vi "Read.vi"(7 "nonEmpty":refnum<k4>, 8 "element in":T3, 10 "parms in":T2={"subchannel"=0, "size (0)"=0, "abort (F)"=FALSE, "timeout"=-1, "ack id (0)"=0, "last elt? (F)"=FALSE, "valid? (T)"=FALSE, "GUID"=""}, 11 "MessengerMCPU in":refnum<class "MessengerMCPU.lvclass">) -> (0 "element out":T3, 1 "wait":bool, 2 "parms out":T1, 3 "MessengerMCPU out":refnum<class "MessengerMCPU.lvclass">)   [LabVIEW 2019, in "MessengerM.lvlib" / "MessengerMCPU.lvclass"]
uses:
  MessengerMCPU.lvclass
  ParmsOut.ctl
  MessengerM.lvlib
  SubChannelCPU/SubChannelCPU.lvclass
  Element.ctl
  ParmsIn.ctl
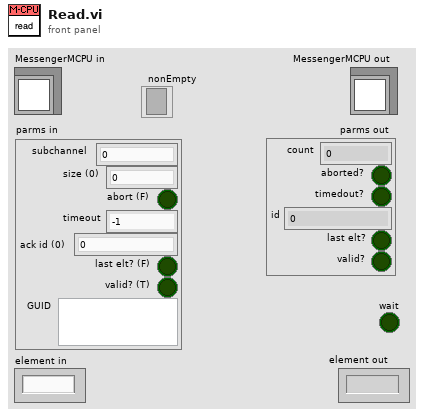
[diagram p1: front panel]
types:
  T1 = typedef "MessengerM.lvlib/ParmsOut.ctl" = cluster{"count":i32, "aborted?":bool, "timedout?":bool, "id":u32, "last elt?":bool, "valid?":bool}
  T2 = typedef "MessengerM.lvlib/ParmsIn.ctl" = cluster{"subchannel":i32, "size (0)":i32, "abort (F)":bool, "timeout":i32, "ack id (0)":u32, "last elt? (F)":bool, "valid? (T)":bool, "GUID":string}
  T3 = typedef "MessengerM.lvlib/Element.ctl" = string
  T4 = cluster{"GUID":string, "sub":refnum<class "SubChannelCPU.lvclass">}[]
  T5 = cluster{"GUID":string, "sub":refnum<class "SubChannelCPU.lvclass">}
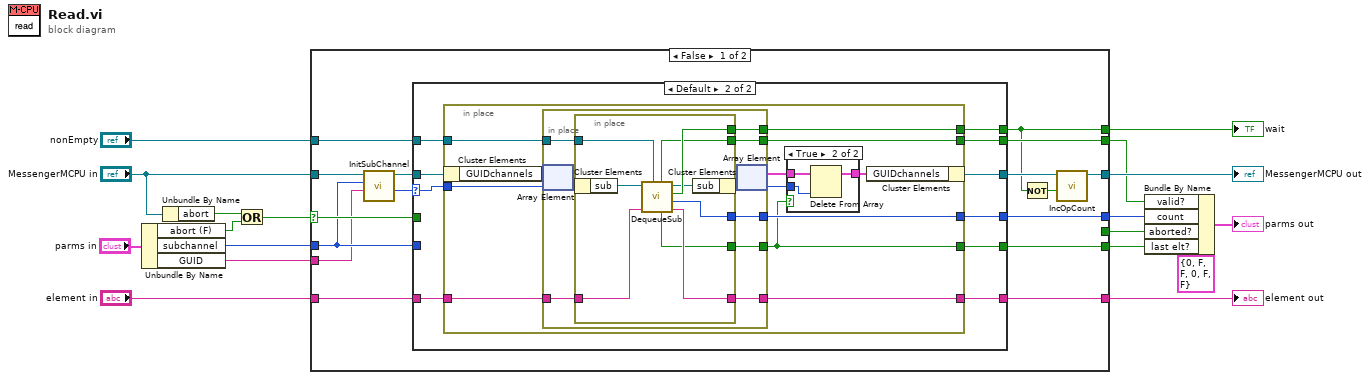
[diagram p0: block diagram]
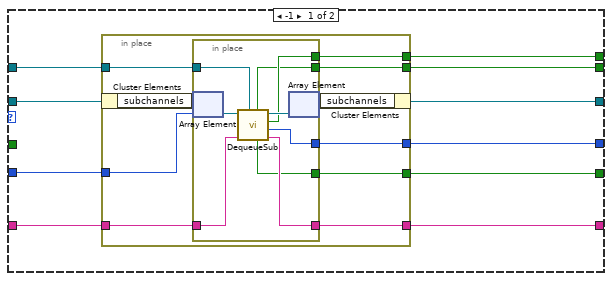
[diagram p2: hidden frame]
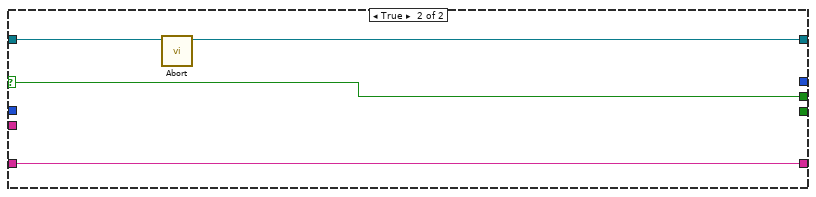
[diagram p4: hidden frame]
diagram:
  n1 = Unbundle By Name("parms in") -> ("abort (F)"=w10:bool, "subchannel"=w9:i32, "GUID"=w1:string)
  n2 = Unbundle By Name("MessengerMCPU in") -> ("abort"=w16:bool)
  n3 = Or(x=w16, y=w10) -> (x .or. y?=w17:bool)
  n4 = case shown="False" w17 {
    selector: w17 -> [w33 w109]
    tunnel: "element in" -> [w34 w108]
    tunnel: [w32 w108] -> w15
    tunnel: [w19 _] -> w14
    tunnel: "MessengerMCPU in" -> [w31 w111]
    tunnel: "nonEmpty" -> [w29 _]
    tunnel: w9 -> [w28 _]
    tunnel: [_ w109] -> w6
    tunnel: [w27 _] -> w5
    tunnel: [w20 w110] -> w4
    tunnel: [w26 _] -> w3
    tunnel: [w25 _] -> w2
    tunnel: w1 -> [w24 _]
    frame False {
      n5 = call "InitSubChannel.vi"("GUID"=w24, "subchannel"=w28, "MessengerMCPU in"=w31) -> ("GUIDsubchannel"=w23:i32, "MessengerMCPU out"=w30:refnum<class "MessengerMCPU.lvclass">)  [unwired: 7 in]
      n6 = case shown="Default" w23 {
        selector: w23 -> [_ w65]
        tunnel: w34 -> [w44 w73]
        tunnel: w33 -> [_ _]
        tunnel: [w43 w72] -> w32
        tunnel: [w42 w71] -> w19
        tunnel: w30 -> [w41 w70]
        tunnel: w29 -> [w40 w69]
        tunnel: w28 -> [w39 _]
        tunnel: [w38 w68] -> w27
        tunnel: [w35 w64] -> w21
        tunnel: [w37 w67] -> w26
        tunnel: [w36 w66] -> w25
        frame -1 {
          n7 = in-place {
            in-place-border: [w54] -> w42
            in-place-border: [w53] -> w38
            in-place-border: w39 -> [w50]
            in-place-border: w44 -> [w49]
            in-place-border: [w48] -> w43
            in-place-border: w40 -> [w47]
            in-place-border: [w46] -> w37
            in-place-border: [w45] -> w36
            n8 = in-place-cluster #1(w41) -> ("subchannels"=w52:refnum<class "SubChannelCPU.lvclass">[])
            n9 = in-place {
              in-place-border: [w59] -> w54
              in-place-border: [w58] -> w53
              in-place-border: w49 -> [w61]
              in-place-border: [w60] -> w48
              in-place-border: w47 -> [w57]
              in-place-border: [w56] -> w46
              in-place-border: [w55] -> w45
              n10 = in-place-array #2(w52, w50) -> (w63:refnum<class "SubChannelCPU.lvclass">)
              n11 = call-dynamic "DequeueSub.vi"("nonEmpty"=w57, "element in"=w61, "SubChannel in"=w63) -> ("element out"=w60:T3, "count"=w58:i32, "wait"=w59:bool, "SubChannel out"=w62:refnum<class "SubChannelCPU.lvclass">, "last element?"=w56:bool, "valid?"=w55:bool)  [unwired: 3 in]
              n12 = in-place-array #2(w62) -> (w51:refnum<class "SubChannelCPU.lvclass">[])  [unwired: 1 out]
            }
            n13 = in-place-cluster #1("subchannels"=w51) -> (w35:refnum<class "MessengerMCPU.lvclass">)
          }
        }
        frame Default {
          n14 = in-place {
            in-place-border: [w85] -> w71
            in-place-border: [w84] -> w68
            in-place-border: w65 -> [w81]
            in-place-border: w73 -> [w80]
            in-place-border: [w79] -> w72
            in-place-border: w69 -> [w78]
            in-place-border: [w74] -> w67
            in-place-border: [w77] -> w66
            n15 = in-place-cluster #3(w70) -> ("GUIDchannels"=w83:T4)
            n16 = in-place {
              in-place-border: [w96] -> w85
              in-place-border: [w95] -> w84
              in-place-border: w80 -> [w98]
              in-place-border: [w97] -> w79
              in-place-border: w78 -> [w94]
              in-place-border: [w93] -> w74
              in-place-border: [w92] -> w77
              n17 = in-place-array #4(w83, w81) -> (w91:T5)
              n18 = in-place {
                in-place-border: w98 -> [w107]
                in-place-border: [w106] -> w97
                in-place-border: [w105] -> w96
                in-place-border: [w104] -> w95
                in-place-border: w94 -> [w103]
                in-place-border: [w102] -> w93
                in-place-border: [w101] -> w92
                n19 = in-place-cluster #5(w91) -> ("sub"=w100:refnum<class "SubChannelCPU.lvclass">)
                n20 = call-dynamic "DequeueSub.vi"("nonEmpty"=w103, "element in"=w107, "SubChannel in"=w100) -> ("element out"=w106:T3, "count"=w104:i32, "wait"=w105:bool, "SubChannel out"=w99:refnum<class "SubChannelCPU.lvclass">, "last element?"=w102:bool, "valid?"=w101:bool)  [unwired: 3 in]
                n21 = in-place-cluster #5("sub"=w99) -> (w90:T5)
              }
              n22 = in-place-array #4(w90) -> (w82:T4, w75:i32)
            }
            n23 = case shown="True" w74 {
              tunnel: w82 -> [w86 w89]
              tunnel: [w86 w88] -> w76
              tunnel: w75 -> [_ w87]
              frame False {
              }
              frame True {
                n24 = Delete From Array(array=w89, index=w87) -> (array with subset deleted=w88:T4)  [unwired: 1 in, 1 out]
              }
            }
            n25 = in-place-cluster #3("GUIDchannels"=w76) -> (w64:refnum<class "MessengerMCPU.lvclass">)
          }
        }
      }
      n26 = Not(x=w19) -> (.not. x?=w22:bool)
      n27 = call-dynamic "IncOpCount.vi"("inc?"=w22, "MessengerMCPU in"=w21) -> ("MessengerMCPU out"=w20:refnum<class "MessengerMCPU.lvclass">)  [unwired: 9 in]
    }
    frame True {
      n28 = call-dynamic "Abort.vi"("MessengerMCPU in"=w111) -> ("MessengerMCPU out"=w110:refnum<class "MessengerMCPU.lvclass">)  [unwired: 10 in]
    }
  }
  "MessengerMCPU out" <- w4
  "element out" <- w15
  "wait" <- w14
  n29 = Bundle By Name(cluster=T1 {"count"=0, "aborted?"=FALSE, "timedout?"=FALSE, "id"=0, "last elt?"=FALSE, "valid?"=FALSE} ("parms out"), "valid?"=w2, "count"=w5, "aborted?"=w6, "last elt?"=w3) -> (→"parms out":T1)
